vi "Facade.vi"(0 "Data In":T5, 2 "Display State In":T2, 3 "Container State":T4) -> (6 "Data Out":T5, 7 "Display State Out":T2, 8 "Action":T1)   [LabVIEW 2015, in "KPropertyTable.xctl"]
uses:
  KPropertyTable.xctl
  Data.vi
  RowData.ctl
  DataType.ctl
  <vilib>/_xctls/Container State.ctl
  State.vi
  <vilib>/_xctls/Action.ctl
  <vilib>/Utility/miscctls.llb/LVRowAndColumnTypeDef.ctl
  <vilib>/_xctls/XControlSupport.lvlib
panel:
  in  "Ring":u16(ring)
  in  "Table":i32(listbox)
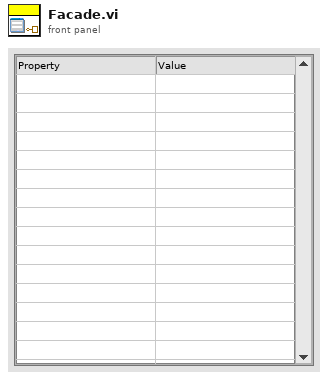
[diagram p1: front panel]
types:
  T1 = typedef "XControlSupport.lvlib/Action.ctl" = cluster{"Data Changed?":bool, "State Changed?":bool, "Action Name":string}
  T2 = typedef "KPropertyTable.xctl/State.vi" = cluster{"show categories":bool, "table":refnum<vi>, "items":i32[], "enum row":i32, "edit type":T3, "edit row":i32, "max rows":i32, "scrollbar":bool}
  T3 = typedef "KPropertyTable.xctl/DataType.ctl" = enum16{"String", "Enum", "Int", "Double", "Boolean", "Ring", "Formula"}
  T4 = typedef "XControlSupport.lvlib/Container State.ctl" = cluster{"Indicator?":bool, "Run Mode?":bool, " Refnum":refnum<vi>}
  T5 = typedef "KPropertyTable.xctl/Data.vi" = T6[]
  T6 = typedef "KPropertyTable.xctl/RowData.ctl" = cluster{"Name":string, "Type":T3, "Category":string, "Strings":string[], "Value":string}
  T7 = typedef "LVRowAndColumnTypeDef.ctl" = cluster{"Row":i32, "Column":i32}
  T8 = typedef "LVPoint32TypeDef.ctl" = cluster{"Horizontal":i32, "Vertical":i32}
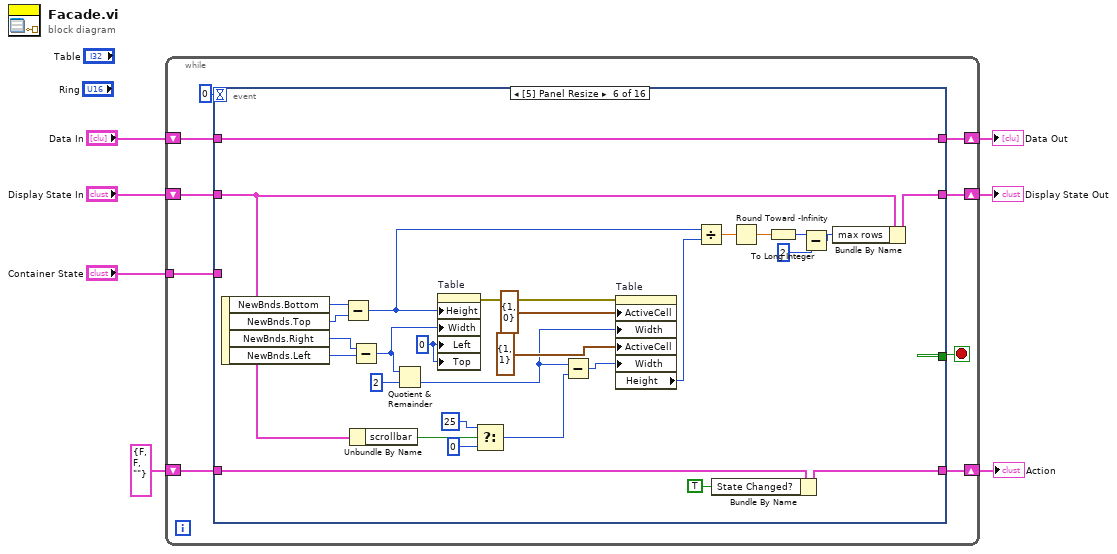
[diagram p0: block diagram]
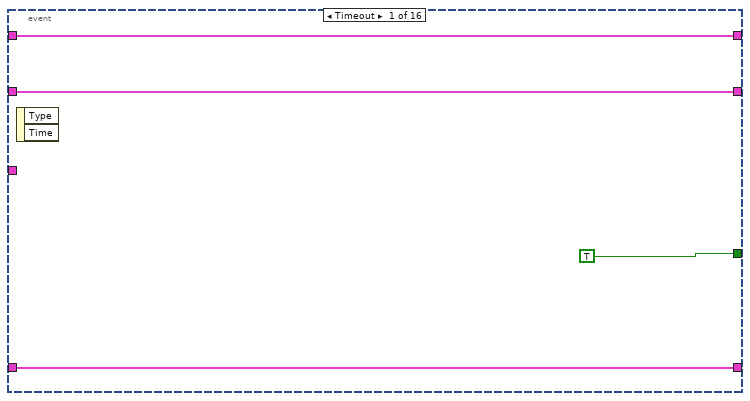
[diagram p2: hidden frame]
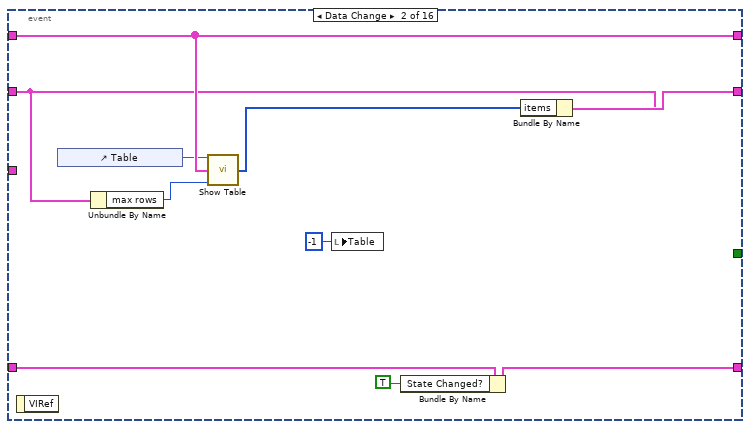
[diagram p3: hidden frame]
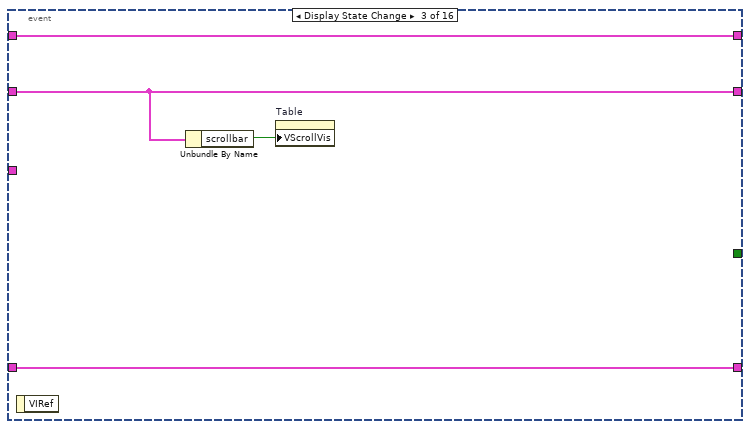
[diagram p4: hidden frame]
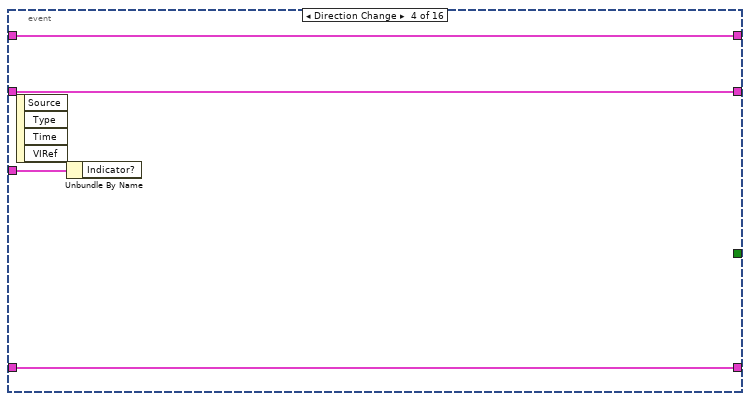
[diagram p5: hidden frame]
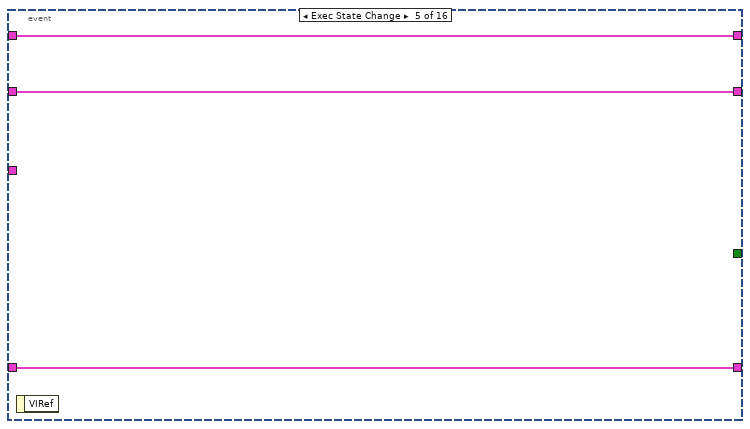
[diagram p6: hidden frame]
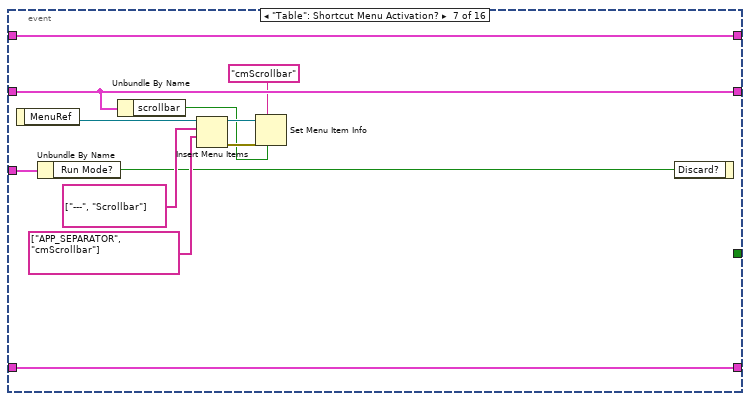
[diagram p7: hidden frame]
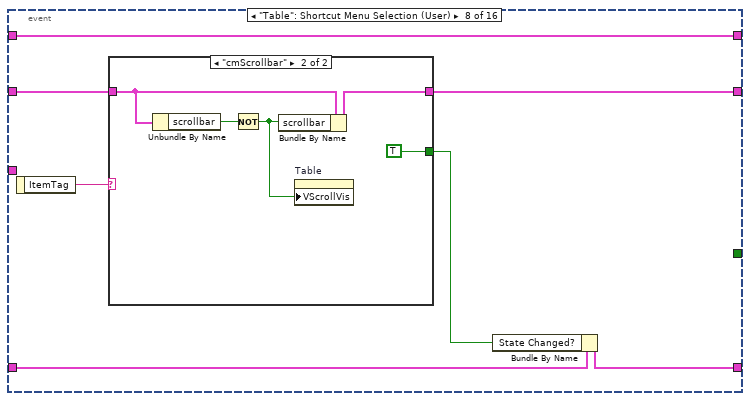
[diagram p8: hidden frame]
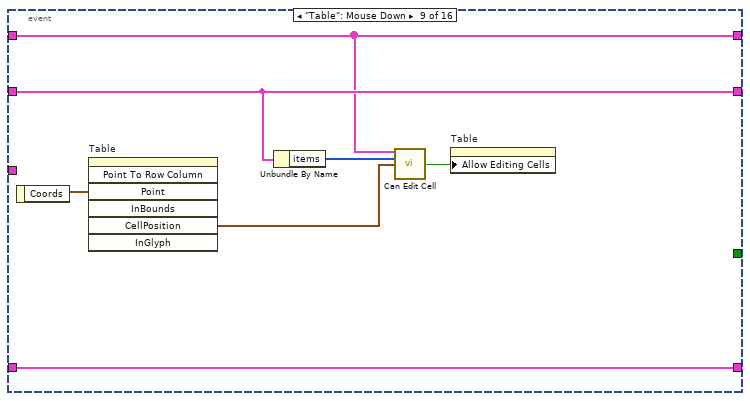
[diagram p10: hidden frame]
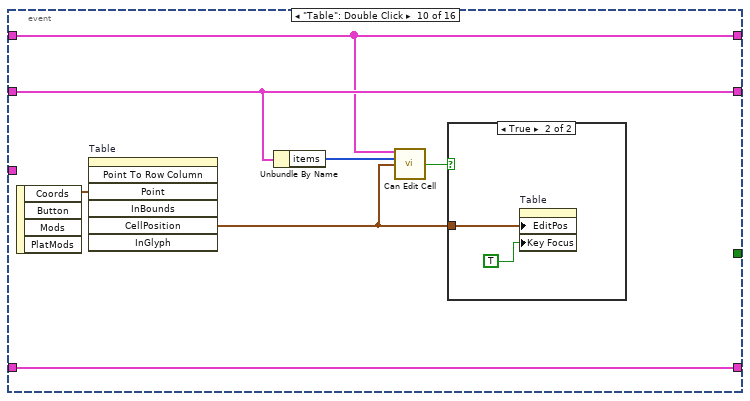
[diagram p11: hidden frame]
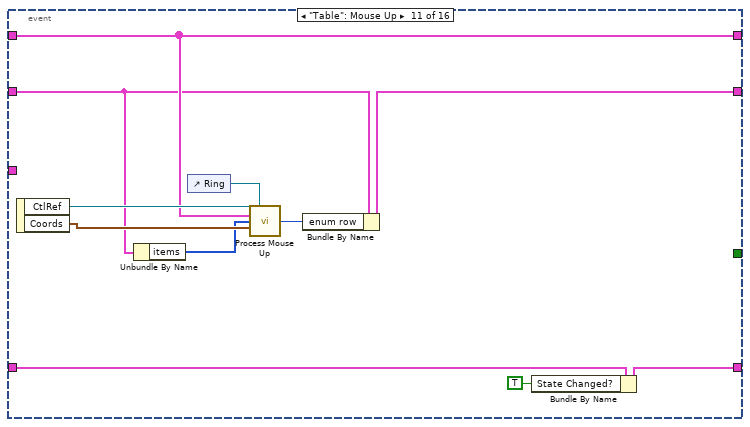
[diagram p13: hidden frame]
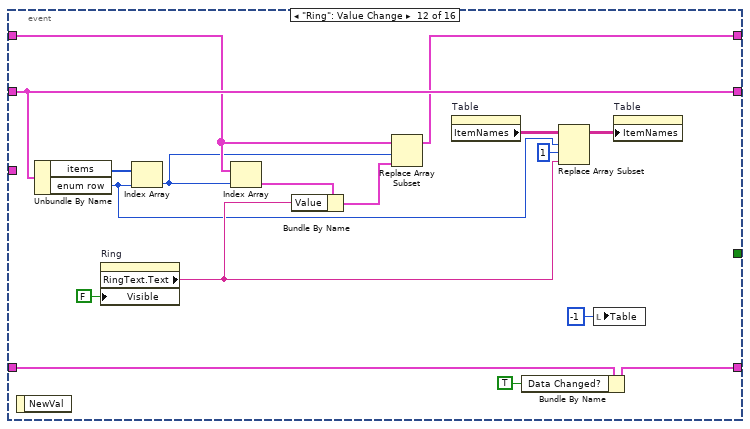
[diagram p14: hidden frame]
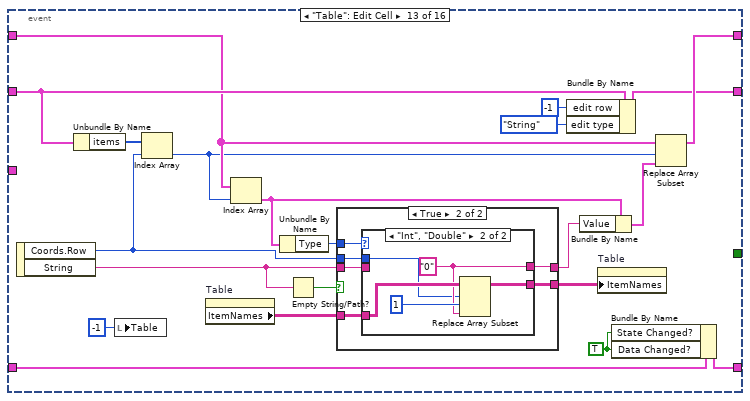
[diagram p15: hidden frame]
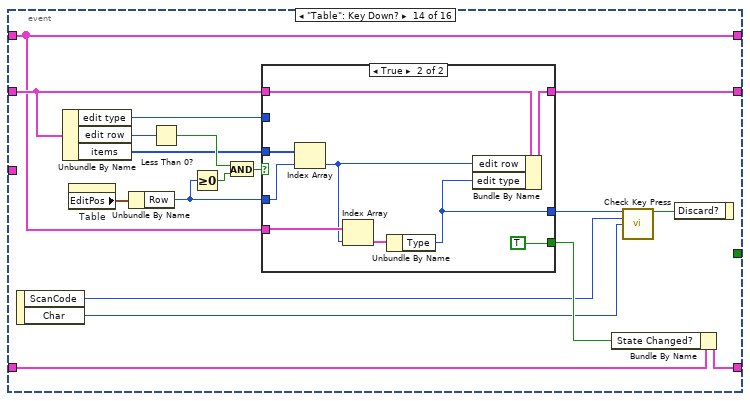
[diagram p18: hidden frame]
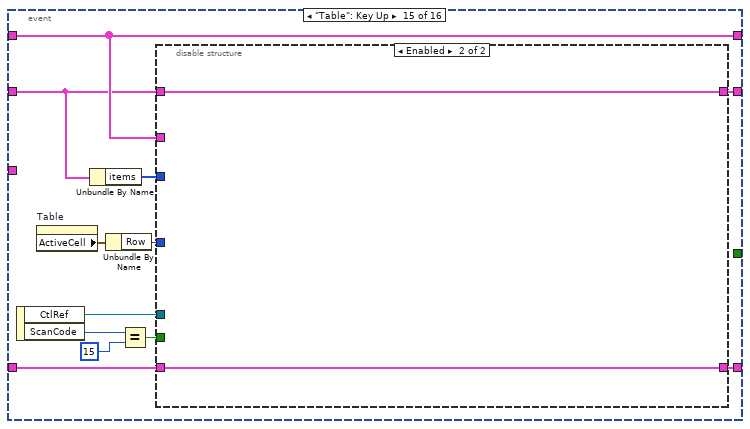
[diagram p20: hidden frame]
diagram:
  n1 = while {
    shift-right: [w15] -> w4
    shift-left: "Display State In" -> [w16]
    tunnel: "Container State" -> [w12]
    shift-right: [w10] -> w7
    shift-left: "Data In" -> [w11]
    shift-right: [w8] -> w2
    shift-left: T1 {"Data Changed?"=FALSE, "State Changed?"=FALSE, "Action Name"=""} ("Action") -> [w9]
    stop <- w14 stop-if-true
    n2 = event shown="[5] Panel Resize" {
      selector: _ -> [_ _ _ _ _ _ _ _ _ _ _ _ _ _ _ _]
      dyn-events: _ -> [_ _ _ _ _ _ _ _ _ _ _ _ _ _ _ _]
      timeout: 0 -> [_ _ _ _ _ _ _ _ _ _ _ _ _ _ _ _]
      tunnel: w16 -> [w18 w24 w32 w37 w41 w46 w73 w86 w100 w107 w117 w138 w159 w188 w208 w271]
      tunnel: [w18 w28 w32 w37 w41 w56 w73 w85 w100 w107 w115 w138 w151 w187 w207 w271] -> w15
      tunnel: [TRUE _ _ _ _ _ _ _ _ _ _ _ _ _ _ _] -> w14
      tunnel: w12 -> [_ _ _ w38 _ _ w77 _ _ _ _ _ _ _ _ _]
      tunnel: w11 -> [w17 w29 w34 w36 w40 w70 w82 w89 w98 w105 w119 w135 w157 w176 w210 w270]
      tunnel: [w17 w29 w34 w36 w40 w70 w82 w89 w98 w105 w119 w134 w156 w176 w210 w270] -> w10
      tunnel: [w19 w26 w33 w35 w39 w55 w81 w84 w102 w109 w113 w132 w155 w186 w205 w269] -> w8
      tunnel: w9 -> [w19 w30 w33 w35 w39 w69 w81 w88 w102 w109 w122 w139 w160 w193 w206 w269]
      event Timeout {
        n3 = event-data() -> ()  [unwired: 1 in, 2 out]
      }
      event Data Change {
        n4 = event-data() -> ()  [unwired: 1 in, 1 out]
        n5 = control-ref of="Table"() -> (w22:refnum<vi>)
        n6 = Unbundle By Name(w24) -> ("max rows"=w23:i32)
        n7 = call "Show Table.vi"("Table"=w22, "Data"=w29, "max rows"=w23) -> ("items"=w27:i32[])  [unwired: 12 in]
        n8 = local write "Table"(-1 ("Table")) -> ()
        n9 = Bundle By Name(cluster=w30, "State Changed?"=TRUE) -> (w26:T1)
        n10 = Bundle By Name(cluster=w24, "items"=w27) -> (w28:T2)
      }
      event Display State Change {
        n11 = event-data() -> ()  [unwired: 1 in, 1 out]
        n12 = Unbundle By Name(w32) -> ("scrollbar"=w31:bool)
        n13 = property on="Table" class="MCListbox (strict)"("VScrollVis"=w31) -> ()  [unwired: 2 in, 2 out]
      }
      event Direction Change {
        n14 = event-data() -> ()  [unwired: 1 in, 4 out]
        n15 = Unbundle By Name(w38) -> ()  [unwired: 1 out]
      }
      event Exec State Change {
        n16 = event-data() -> ()  [unwired: 1 in, 1 out]
      }
      event Panel Resize {
        w58 = 0 ("Position:Left")
        n17 = event-data() -> ("NewBnds.Bottom"=w68:i16, "NewBnds.Top"=w67:i16, "NewBnds.Right"=w66:i16, "NewBnds.Left"=w65:i16)  [unwired: 1 in]
        n18 = Subtract(x=w68, y=w67) -> (x-y=w53:i16)
        n19 = Unbundle By Name(w46) -> ("scrollbar"=w45:bool)
        n20 = Subtract(x=w66, y=w65) -> (x-y=w64:i16)
        n21 = Quotient & Remainder(x=w64, y=i16 2) -> (floor(x/y)=w59:i16)  [unwired: 1 out]
        n22 = property on="Table" class="MCListbox (strict)"("Height"=w53, "Width"=w64, "Left"=w58, "Top"=w58) -> (error out=w62:errorcluster)  [unwired: 2 in, 1 out]
        n23 = Select(t=i16 25 ("y"), s=w45, f=i16 0) -> (s? t:f=w42:i16)
        n24 = Subtract(x=w59, y=w42) -> (x-y=w57:i16)
        n25 = property on="Table" class="MCListbox (strict)"(error in=w62, "ActiveCell"=T7 {"Row"=1, "Column"=0} ("Active Cell:Active Cell"), "Width"=w59, "ActiveCell"=T7 {"Row"=1, "Column"=1} ("Active Cell:Active Cell"), "Width"=w57) -> ("Height"=w52:u32)  [unwired: 1 in, 2 out]
        n26 = Divide(x=w53, y=w52) -> (x/y=w51:dbl)
        n27 = Bundle By Name(cluster=w69, "State Changed?"=TRUE) -> (w55:T1)
        n28 = Round Toward -Infinity(1:w51) -> (0:w50:dbl)
        n29 = To Long Integer(number=w50) -> (32bit integer=w49:i32)
        n30 = Subtract(x=w49, y=2) -> (x-y=w47:i32)
        n31 = Bundle By Name(cluster=w46, "max rows"=w47) -> (w56:T2)
      }
      event "Table": Shortcut Menu Activation? {
        n32 = event-data() -> ("MenuRef"=w80:refnum<k9>)  [unwired: 1 in]
        n33 = Unbundle By Name(w77) -> ("Run Mode?"=w76:bool)
        n34 = Unbundle By Name(w73) -> ("scrollbar"=w72:bool)
        n35 = Insert Menu Items(7:string[] ["APP_SEPARATOR", "cmScrollbar"] ("item tags"), 8:string[] ["---", "Scrollbar"] ("item names"), 9:w80) -> (0:w75:errorcluster, 3:w74:refnum<k9>)  [unwired: 3 in, 1 out]
        n36 = Set Menu Item Info(6:w72, 7:"cmScrollbar" ("item tag"), 8:w75, 11:w74) -> ()  [unwired: 3 in, 2 out]
        n37 = event-data("Discard?"=w76) -> ()  [unwired: 1 in, 1 out]
      }
      event "Table": Shortcut Menu Selection (User) {
        n38 = event-data() -> ("ItemTag"=w87:string)  [unwired: 1 in]
        n39 = case shown="\"cmScrollbar\"" w87 {
          tunnel: w86 -> [w90 w95]
          tunnel: [w90 w93] -> w85
          tunnel: [_ TRUE] -> w83
          frame "", Default {
          }
          frame "cmScrollbar" {
            n40 = Unbundle By Name(w95) -> ("scrollbar"=w94:bool)
            n41 = Not(x=w94) -> (.not. x?=w91:bool)
            n42 = Bundle By Name(cluster=w95, "scrollbar"=w91) -> (w93:T2)
            n43 = property on="Table" class="MCListbox (strict)"("VScrollVis"=w91) -> ()  [unwired: 2 in, 2 out]
          }
        }
        n44 = Bundle By Name(cluster=w88, "State Changed?"=w83) -> (w84:T1)
      }
      event "Table": Mouse Down {
        n45 = event-data() -> ("Coords"=w101:T8)  [unwired: 1 in]
        n46 = invoke on="Table" class="MCListbox (strict)" method="Point To Row Column"("Point"=w101) -> ("CellPosition"=w97:T7)  [unwired: 6 in, 6 out]
        n47 = Unbundle By Name(w100) -> ("items"=w99:i32[])
        n48 = call "Can Edit Cell.vi"("Rows"=w98, "Items"=w99, "Cell"=w97) -> ("can edit?"=w96:bool)  [unwired: 9 in, 3 out]
        n49 = property on="Table" class="MCListbox (strict)"("Allow Editing Cells"=w96) -> ()  [unwired: 2 in, 2 out]
      }
      event "Table": Double Click {
        n50 = event-data() -> ("Coords"=w108:T8)  [unwired: 1 in, 3 out]
        n51 = invoke on="Table" class="MCListbox (strict)" method="Point To Row Column"("Point"=w108) -> ("CellPosition"=w104:T7)  [unwired: 6 in, 6 out]
        n52 = Unbundle By Name(w107) -> ("items"=w106:i32[])
        n53 = call "Can Edit Cell.vi"("Rows"=w105, "Items"=w106, "Cell"=w104) -> ("can edit?"=w103:bool)  [unwired: 9 in, 3 out]
        n54 = case shown="True" w103 {
          tunnel: w104 -> [_ w110]
          frame False {
          }
          frame True {
            n55 = property on="Table" class="MCListbox (strict)"("EditPos"=w110, "Key Focus"=TRUE) -> ()  [unwired: 2 in, 2 out]
          }
        }
      }
      event "Table": Mouse Up {
        n56 = event-data() -> ("CtlRef"=w121:refnum<vi>, "Coords"=w118:T8)  [unwired: 1 in]
        n57 = Unbundle By Name(w117) -> ("items"=w116:i32[])
        n58 = control-ref of="Ring"() -> (w120:refnum<vi>)
        n59 = call "Process Mouse Up.vi"("Listbox"=w121, "Ring"=w120, "Rows"=w119, "Items"=w116, "Coords"=w118) -> ("row"=w114:i32)  [unwired: 9 in, 1 out]
        n60 = Bundle By Name(cluster=w117, "enum row"=w114) -> (w115:T2)
        n61 = Bundle By Name(cluster=w122, "State Changed?"=TRUE) -> (w113:T1)
      }
      event "Ring": Value Change {
        n62 = event-data() -> ()  [unwired: 1 in, 1 out]
        n63 = Unbundle By Name(w138) -> ("items"=w126:i32[], "enum row"=w124:i32)
        n64 = property on="Ring" class="Ring (strict)"("Visible"=FALSE) -> ("RingText.Text"=w128:string)  [unwired: 2 in, 2 out]
        n65 = Index Array(array=w126, index=w124) -> (element=w125:i32)
        n66 = Index Array(array=w135, index=w125) -> (element=w137:T6)
        n67 = Bundle By Name(cluster=w137, "Value"=w128) -> (w136:T6)
        n68 = Replace Array Subset(array=w135, new element=w136, index=w125) -> (w134:T5)
        n69 = property on="Table" class="MCListbox (strict)"() -> ("ItemNames"=w130:string[][])  [unwired: 2 in, 2 out]
        n70 = Bundle By Name(cluster=w139, "Data Changed?"=TRUE) -> (w132:T1)
        n71 = Replace Array Subset(array=w130, new element=w128, index (row)=w124, index (col)=1 ("disabled index (col)")) -> (w127:string[][])
        n72 = local write "Table"(-1 ("Table")) -> ()
        n73 = property on="Table" class="MCListbox (strict)"("ItemNames"=w127) -> ()  [unwired: 2 in, 2 out]
      }
      event "Table": Edit Cell {
        w152 = TRUE ("Data Changed?")
        n74 = event-data() -> ("Coords.Row"=w143:i32, "String"=w147:string)  [unwired: 1 in]
        n75 = Unbundle By Name(w159) -> ("items"=w154:i32[])
        n76 = local write "Table"(-1 ("Table")) -> ()
        n77 = Index Array(array=w154, index=w143) -> (element=w153:i32)
        n78 = property on="Table" class="MCListbox (strict)"() -> ("ItemNames"=w144:string[][])  [unwired: 2 in, 2 out]
        n79 = Index Array(array=w157, index=w153) -> (element=w149:T6)
        n80 = Unbundle By Name(w149) -> ("Type"=w145:T3)
        n81 = Empty String/Path?(string/path=w147) -> (empty?=w148:bool)
        n82 = case shown="True" w148 {
          tunnel: w147 -> [w162 w166]
          tunnel: [w162 w167] -> w146
          tunnel: w145 -> [_ w168]
          tunnel: w144 -> [w161 w165]
          tunnel: w143 -> [_ w164]
          tunnel: [w161 w163] -> w142
          frame False {
          }
          frame True {
            n83 = case shown="\"Int\", \"Double\"" w168 {
              tunnel: [w170 w173] -> w167
              tunnel: w166 -> [w170 _]
              tunnel: w165 -> [w169 w174]
              tunnel: w164 -> [_ w172]
              tunnel: [w169 w171] -> w163
              frame "String", Default {
              }
              frame "Int", "Double" {
                w173 = "0"
                n84 = Replace Array Subset(array=w174, new element=w173, index (row)=w172, index (col)=1 ("disabled index (col)")) -> (w171:string[][])
              }
            }
          }
        }
        n85 = Bundle By Name(cluster=w159, "edit row"=-1, "edit type"=DataType."String") -> (w151:T2)
        n86 = Bundle By Name(cluster=w149, "Value"=w146) -> (w158:T6)
        n87 = property on="Table" class="MCListbox (strict)"("ItemNames"=w142) -> ()  [unwired: 2 in, 2 out]
        n88 = Bundle By Name(cluster=w160, "State Changed?"=w152, "Data Changed?"=w152) -> (w155:T1)
        n89 = Replace Array Subset(array=w157, new element=w158, index=w153) -> (w156:T5)
      }
      event "Table": Key Down? {
        n90 = event-data() -> ("ScanCode"=w180:i16, "Char"=w179:i16)  [unwired: 1 in]
        n91 = Unbundle By Name(w188) -> ("edit type"=w181:T3, "edit row"=w192:i32, "items"=w189:i32[])
        n92 = property on="Table" class="MCListbox (strict)"() -> ("EditPos"=w191:T7)  [unwired: 2 in, 2 out]
        n93 = Unbundle By Name(w191) -> ("Row"=w183:i32)
        n94 = Less Than 0?(x=w192) -> (x < 0?=w190:bool)
        n95 = Greater Or Equal To 0?(x=w183) -> (x >= 0?=w184:bool)
        n96 = And(x=w190, y=w184) -> (x .and. y?=w185:bool)
        n97 = case shown="True" w185 {
          tunnel: w183 -> [_ w202]
          tunnel: w189 -> [_ w204]
          tunnel: w188 -> [w195 w203]
          tunnel: [w195 w198] -> w187
          tunnel: w176 -> [_ w201]
          tunnel: [_ TRUE] -> w182
          tunnel: [w194 w196] -> w178
          tunnel: w181 -> [w194 _]
          frame False {
          }
          frame True {
            n98 = Index Array(array=w204, index=w202) -> (element=w200:i32)
            n99 = Index Array(array=w201, index=w200) -> (element=w199:T6)
            n100 = Unbundle By Name(w199) -> ("Type"=w196:T3)
            n101 = Bundle By Name(cluster=w203, "edit row"=w200, "edit type"=w196) -> (w198:T2)
          }
        }
        n102 = Bundle By Name(cluster=w193, "State Changed?"=w182) -> (w186:T1)
        n103 = call "Check Key Press.vi"("Type"=w178, "ScanCode"=w180, "Char"=w179) -> ("Discard?"=w177:bool)  [unwired: 12 in]
        n104 = event-data("Discard?"=w177) -> ()  [unwired: 1 in, 1 out]
      }
      event "Table": Key Up {
        n105 = event-data() -> ("CtlRef"=w209:refnum<vi>, "ScanCode"=w216:i16)  [unwired: 1 in]
        n106 = property on="Table" class="MCListbox (strict)"() -> ("ActiveCell"=w213:T7)  [unwired: 2 in, 2 out]
        n107 = Unbundle By Name(w208) -> ("items"=w211:i32[])
        n108 = Unbundle By Name(w213) -> ("Row"=w212:i32)
        n109 = Equal?(x=w216, y=i16 15) -> (x = y?=w214:bool)
        n110 = disable-structure shown="Enabled" {
          disable-tunnel: w214 -> [w225 _]
          disable-tunnel: w212 -> [w224 _]
          disable-tunnel: w211 -> [w223 _]
          disable-tunnel: w210 -> [w222 _]
          disable-tunnel: w209 -> [w221 _]
          disable-tunnel: w208 -> [w220 w267]
          disable-tunnel: [w219 w267] -> w207
          disable-tunnel: w206 -> [w218 w266]
          disable-tunnel: [w217 w266] -> w205
          frame Disabled {
            n111 = case shown="True" w225 {
              tunnel: w224 -> [_ w241]
              tunnel: w223 -> [_ w240]
              tunnel: w222 -> [_ w239]
              tunnel: w221 -> [_ w236]
              tunnel: w220 -> [w227 w231]
              tunnel: [w227 w230] -> w219
              tunnel: w218 -> [w226 w229]
              tunnel: [w226 w228] -> w217
              frame False {
              }
              frame True {
                n112 = while {
                  tunnel: w240 -> [w264]
                  shift-right: [w258] -> w233
                  shift-left: w241 -> [w265]
                  tunnel: [w257] -> w238
                  stop <- w259 stop-if-true
                  n113 = Increment(x=w265) -> (x+1=w261:i32)
                  n114 = Array Size(array=w264) -> (size(s)=w263:i32)
                  n115 = Equal?(x=w263, y=w261) -> (x = y?=w262:bool)
                  n116 = Select(t=0, s=w262, f=w261) -> (s? t:f=w258:i32)
                  n117 = Index Array(array=w264, index=w258) -> (element=w257:i32)
                  n118 = Greater Or Equal To 0?(x=w257) -> (x >= 0?=w259:bool)
                }
                n119 = Index Array(array=w239, index=w238) -> (element=w235:T6)
                n120 = Unbundle By Name(w235) -> ("Type"=w237:T3)
                n121 = Bundle("Row"=w233, 1) -> (w232:cluster{"Row":i32, i32})  [unwired: 1 in]
                n122 = case shown="\"Enum\"" w237 {
                  tunnel: w236 -> [_ w256]
                  tunnel: w235 -> [_ w254]
                  tunnel: w232 -> [w244 w251]
                  tunnel: w231 -> [w243 w253]
                  tunnel: [w243 w252] -> w230
                  tunnel: w229 -> [w242 w249]
                  tunnel: [w242 w248] -> w228
                  frame "String", Default {
                    n123 = property on="Table" class="MCListbox (strict)"("EditPos"=w244, "ActiveCell"=w244, "Key Focus"=TRUE) -> ()  [unwired: 2 in, 2 out]
                  }
                  frame "Enum" {
                    n124 = control-ref of="Ring"() -> (w255:refnum<vi>)
                    n125 = Unbundle(w251) -> ("Row"=w250:i32)  [unwired: 1 out]
                    n126 = call "Show Ring.vi"("Listbox"=w256, "Ring"=w255, "item"=w254, "cell"=w251) -> ()  [unwired: 11 in, 1 out]
                    n127 = Decrement(x=w250) -> (x-1=w246:i32)
                    n128 = Bundle By Name(cluster=w249, "State Changed?"=TRUE) -> (w248:T1)
                    n129 = Bundle By Name(cluster=w253, "enum row"=w246) -> (w252:T2)
                  }
                }
              }
            }
          }
          frame Enabled {
          }
        }
      }
      event Mouse Leave {
        n130 = event-data() -> ()  [unwired: 1 in, 1 out]
        n131 = property on="Ring" class="Ring (strict)"("Visible"=FALSE) -> ()  [unwired: 2 in, 2 out]
      }
    }
  }
  "Display State Out" <- w4
  "Data Out" <- w7
  "Action" <- w2
